vi "AddSensor.vi"(10 "Connection In":refnum<k7>) -> (2 "OK Button 2":bool)   [LabVIEW 2026]
panel:
  in  "Alarm Limit":i32
  in  "Asset":u16(ring) items=["dg1"=1, "dg2"=7, "dg3"=8, "dg4"=9, "ah1"=10]
  in  "Cancel Button":bool
  in  "OK Button":bool
  in  "Type":u16(ring) items=["Temp"=1, "RPM"=2]
  in  "Sampling time [ms]":dbl
  in  "Unit":string
  in  "Model":string
  in  "Manufacturer":string
  # "New Sensor"
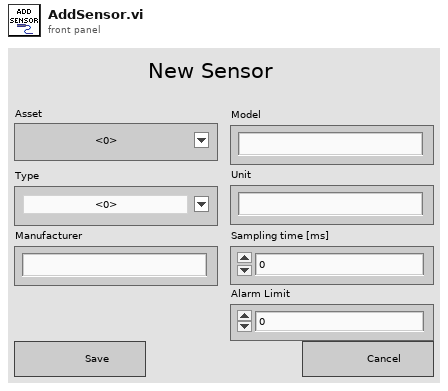
[diagram p1: front panel]
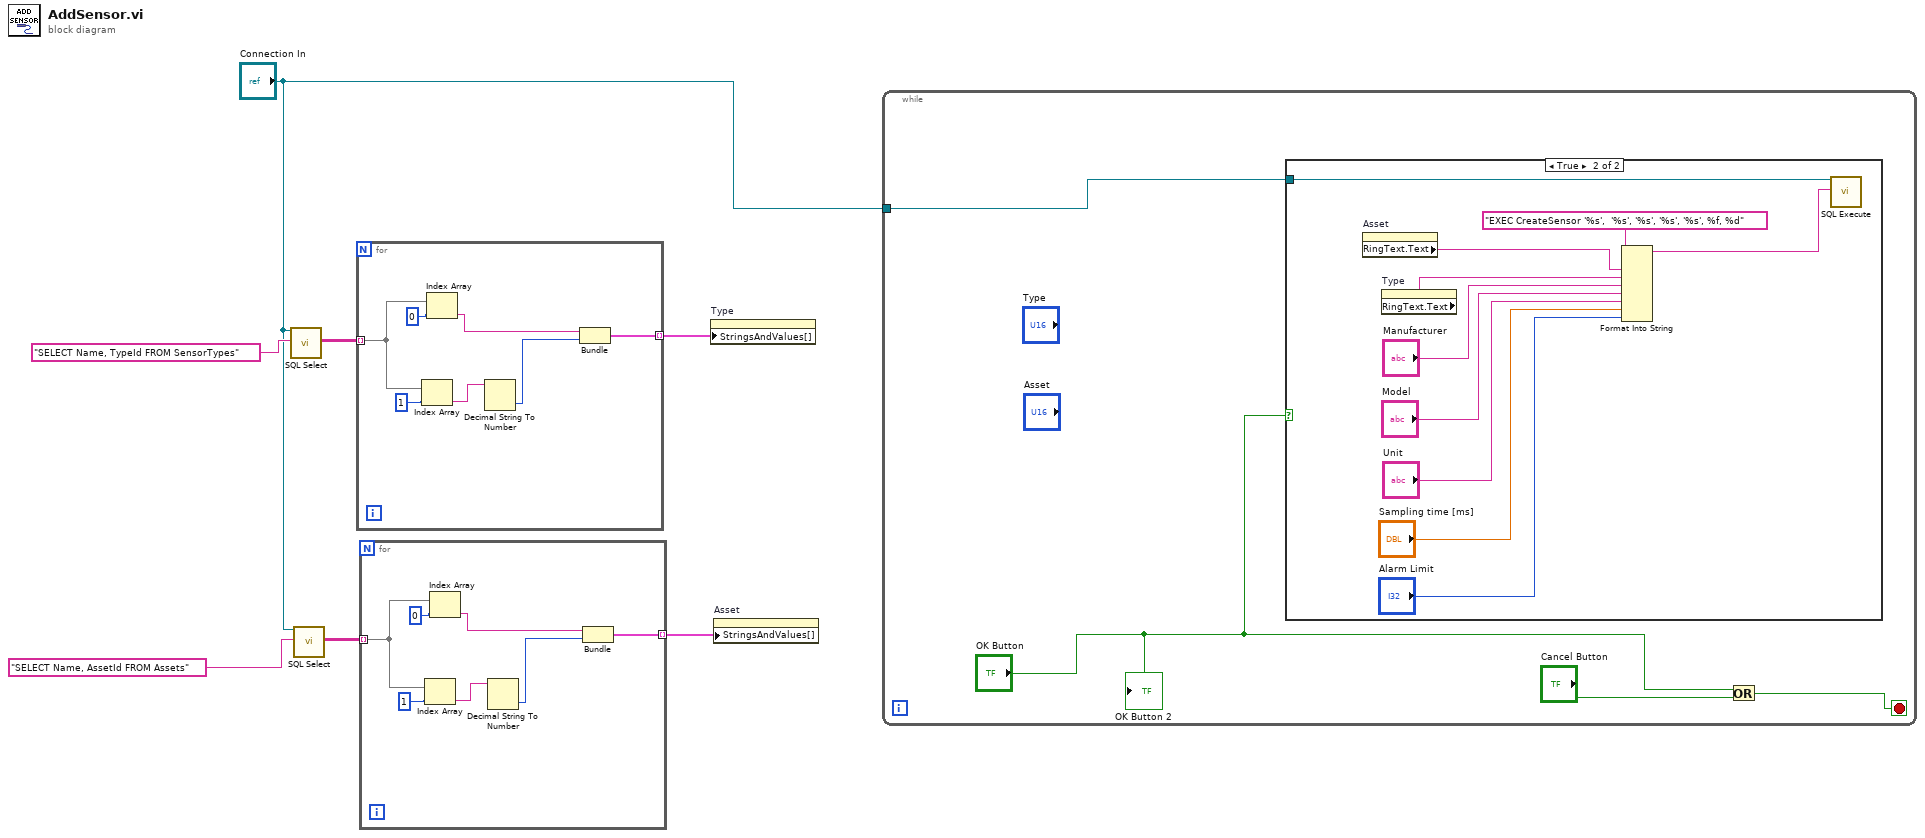
[diagram p0: block diagram]
diagram:
  n1 = call <vilib>:"SQL Select.vi"("Connection In"="Connection In", "SQL Query"="SELECT Name, TypeId FROM SensorTypes") -> ("Data"=w6:string[][])  [unwired: 15 in, 2 out]
  n2 = call <vilib>:"SQL Select.vi"("Connection In"="Connection In", "SQL Query"="SELECT Name, AssetId FROM Assets") -> ("Data"=w4:string[][])  [unwired: 15 in, 2 out]
  n3 = for {
    tunnel: w6 -> [w12] mode=indexing
    tunnel: [w8] -> w5 mode=indexing
    n4 = Index Array "Index Array"(array=w12, index=1) -> (element=w10:string)
    n5 = Index Array "Index Array"(array=w12, index=0) -> (element=w11:string)
    n6 = Decimal String To Number(string=w10) -> (number=w9:i32)  [unwired: 2 in, 1 out]
    n7 = Bundle("String"=w11, w9) -> (w8:cluster{"String":string, i32})  [unwired: 1 in]
  }
  n8 = for {
    tunnel: w4 -> [w19] mode=indexing
    tunnel: [w15] -> w3 mode=indexing
    n9 = Index Array "Index Array"(array=w19, index=1) -> (element=w17:string)
    n10 = Index Array "Index Array"(array=w19, index=0) -> (element=w18:string)
    n11 = Decimal String To Number(string=w17) -> (number=w16:i32)  [unwired: 2 in, 1 out]
    n12 = Bundle("String"=w18, w16) -> (w15:cluster{"String":string, i32})  [unwired: 1 in]
  }
  n13 = property on="Type" class="Ring (strict)"("StringsAndValues[]"=w5) -> ()  [unwired: 2 in, 2 out]
  n14 = property on="Asset" class="Ring (strict)"("StringsAndValues[]"=w3) -> ()  [unwired: 2 in, 2 out]
  n15 = while {
    tunnel: "Connection In" -> [w23]
    stop <- w25 stop-if-true
    n16 = case shown="True" "OK Button" {
      tunnel: w23 -> [_ w35]
      frame False {
      }
      frame True {
        n17 = property on="Asset" class="Ring (strict)"() -> ("RingText.Text"=w28:string)  [unwired: 2 in, 2 out]
        n18 = property on="Type" class="Ring (strict)"() -> ("RingText.Text"=w27:string)  [unwired: 2 in, 2 out]
        n19 = Format Into String(format string="EXEC CreateSensor '%s',  '%s', '%s', '%s', '%s', %f, %d", w28, w27, "Manufacturer", "Model", "Unit", "Sampling time [ms]", "Alarm Limit") -> (resulting string=w33:string)  [unwired: 2 in, 1 out]
        n20 = call <vilib>:"SQL Execute.vi"("Connection In"=w35, "SQL Query"=w33) -> ()  [unwired: 16 in, 2 out]
      }
    }
    n21 = Or(x="OK Button", y="Cancel Button") -> (x .or. y?=w25:bool)
    "OK Button 2" <- "OK Button"
  }
